vi "Create Sort Key.vi"(8 "error in (no error)":errorcluster, 10 "Input Channels":T1[](array[typedef]) format="%.0x", 11 "Custom Device Ref in":T1 format="%.0x") -> (0 "error out":errorcluster, 3 "Key":enum16{"SimTC", "Calibration", "VO", "CO"}[](array[ring]))   [LabVIEW 2011, in "Simulated Thermocouple Custom Device.lvlib"]
uses:
  Simulated Thermocouple Custom Device.lvlib
  <vilib>/NI Veristand/Custom Device API/Custom Device Item Ref.ctl
  <vilib>/NI Veristand/Custom Device Tools/Custom Device Utility Library/Custom Device Utility Library.lvlib
  <vilib>/NI Veristand/Custom Device API/Custom Device API.lvlib
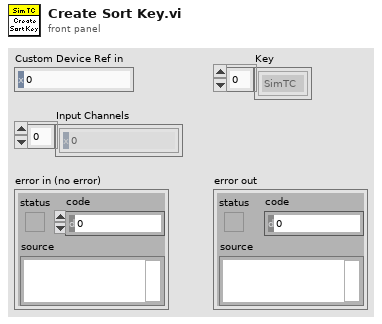
[diagram p1: front panel]
types:
  T1 = typedef "Custom Device API.lvlib/Custom Device Item Ref.ctl" = u64
  T2 = typedef "Custom Device API.lvlib/Custom Device Item Info.ctl" = cluster{"Name":string, "Is Channel":bool, "GUID":string}
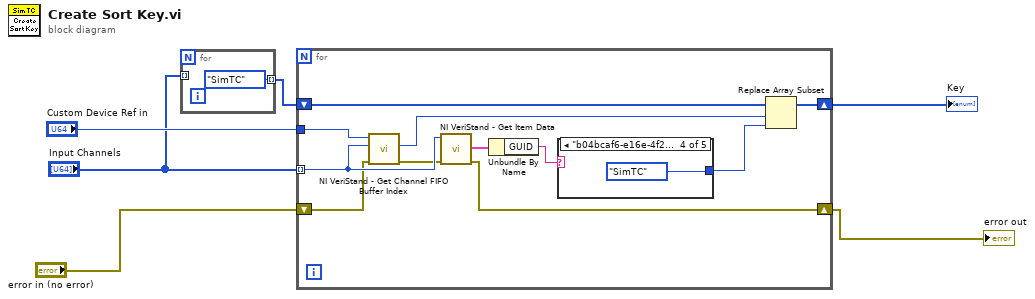
[diagram p0: block diagram]
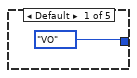
[diagram p2: hidden frame]
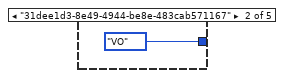
[diagram p3: hidden frame]
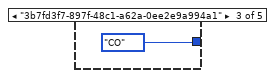
[diagram p4: hidden frame]
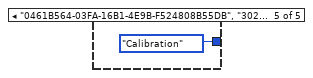
[diagram p5: hidden frame]
diagram:
  n1 = for {
    tunnel: [enum16{"SimTC", "Calibration", "VO", "CO"}."SimTC" ("Channel Type")] -> w2 mode=indexing
    tunnel: "Input Channels" -> [_] mode=indexing
  }
  n2 = for {
    tunnel: "Input Channels" -> [w15] mode=indexing
    shift-right: [w10] -> w6
    shift-left: w2 -> [w16]
    tunnel: "Custom Device Ref in" -> [w18]
    shift-right: [w8] -> w5
    shift-left: "error in (no error)" -> [w9]
    n3 = call <vilib>:"NI VeriStand - Get Channel FIFO Buffer Index.vi"("error in"=w9, "Channel Ref"=w15, "Device Ref in"=w18) -> ("error out"=w14:errorcluster, "Channel FIFO Buffer Index"=w17:i32)  [unwired: 4 in, 3 out]
    n4 = call <vilib>:"NI VeriStand - Get Item Data.vi"("error in (no error)"=w14, "Item Ref in"=w15) -> ("error out"=w8:errorcluster, "Item Info"=w13:T2)  [unwired: 6 in, 2 out]
    n5 = Unbundle By Name(w13) -> ("GUID"=w12:string)
    n6 = case shown="\"b04bcaf6-e16e-4f2b-a421-09dcc5771ba7\"" w12 {
      tunnel: [enum16{"SimTC", "Calibration", "VO", "CO"}."VO" ("Channel Type") enum16{"SimTC", "Calibration", "VO", "CO"}."VO" ("Channel Type") enum16{"SimTC", "Calibration", "VO", "CO"}."CO" ("Channel Type") enum16{"SimTC", "Calibration", "VO", "CO"}."SimTC" ("Channel Type") enum16{"SimTC", "Calibration", "VO", "CO"}."Calibration" ("Channel Type")] -> w11
      frame Default {
      }
      frame "31dee1d3-8e49-4944-be8e-483cab571167" {
      }
      frame "3b7fd3f7-897f-48c1-a62a-0ee2e9a994a1" {
      }
      frame "b04bcaf6-e16e-4f2b-a421-09dcc5771ba7" {
      }
      frame "0461B564-03FA-16B1-4E9B-F524808B55DB", "3027efba-c0b5-45a3-8ca2-970824ba31f4", "B4E1BD10-0157-C0E4-D269-AFE2C6056A58" {
      }
    }
    n7 = Replace Array Subset(array=w16, new element=w11, index=w17) -> (w10:enum16{"SimTC", "Calibration", "VO", "CO"}[])
  }
  "Key" <- w6
  "error out" <- w5
